vi "Aquire HackRF.vi"() -> ()   [LabVIEW 2020]
uses:
  <vilib>/sound2/lvsound2.llb/Sampling Mode.ctl
  <vilib>/sound2/lvsound2.llb/Sound Data Format.ctl
  <vilib>/Analysis/2dsp.llb/Decimate (single shot, DBL).vi
  <vilib>/addons/Adaptive Filters/Create/AFT Create FIR LMS (Real).vi
  <vilib>/addons/Digital Filter Design/Design.llb/DFD IIR Notch Peak Design by Q.vi
  <vilib>/sound2/lvsound2.llb/Sound Output Write (DBL Single).vi
  <vilib>/Analysis/3filter.llb/Butterworth Filter (CDB).vi
  <vilib>/measure/maresamp.llb/Resample Waveform (single shot).vi
  <vilib>/measure/maspectr.llb/FFT Spectrum (Mag-Phase) for 1 Chan.vi
  <vilib>/Analysis/3filter.llb/Butterworth Filter (DBL).vi
  <vilib>/Analysis/3filter.llb/IIR Filter (DBL).vi
  <vilib>/addons/Adaptive Filters/Processing/AFT Filter Signal and Update Coefficients (Real, Array).vi
  HRF_Device/HRF_Device.lvclass
  <vilib>/measure/NI_MAPro.lvlib
  <vilib>/Analysis/NI_AALBase.lvlib
  <vilib>/measure/NI_MABase.lvlib
  <vilib>/Analysis/NI_AALPro.lvlib
  <vilib>/addons/Adaptive Filters/NI_AdaptiveFilter.lvlib
  <vilib>/addons/Digital Filter Design/NI_DigFilterLicensed.lvlib
panel:
  in  "averaging parameters":T1={"averaging mode"=enum."Peak hold", "weighting mode"=enum."Linear", "number of averages"=10} {"number of averages" min=1}
  in  "view":T2={"dB On (F)"=TRUE, "unwrap phase (F)"=FALSE, "convert to degree (F)"=FALSE}
  in  "Enum 2":T3(ring)
  in  "sample rate (S/s)":enum16{"11025", "22050", "44100", "8000"}(ring)=enum."44100"
  in  "bits per sample":enum16{"8 bit", "16 bit"}(ring)=enum."16 bit"
  in  "channel":enum16{"mono", "stereo"}(ring)=enum."stereo"
  in  "scale":dbl=2.5 format="%#_13g"
  in  "cutoff freq":dbl=50000.0
  in  "order":i32=5
  in  "Enum":T3(ring)
  in  "Sample rate":dbl=44100.0
  in  "Interpolation mode":T4(ring)=enum."FIR filter"
  in  "Interpolation mode":T4(ring)=enum."FIR filter"
  in  "FIR filter specifications":T5={"alias rejection"=80.0, "norm bandwdt"=0.45}
  in  "FIR filter specifications":T5={"alias rejection"=40.0, "norm bandwdt"=0.45}
  in  "Resample":bool
  in  "Volume":dbl(knob)=0.76 step=0.01 scale=0.0..2.0
  in  "Order":i32=5
  in  "high cutoff freq: fh 2":dbl=100000.0 format="%0.2f"
  in  "filter input":bool=TRUE
  in  "averaging":bool=TRUE
  out "decimating factor":i32=5
  in  "Cutoff freq":dbl=50000.0 format="%#_13g"
  in  "Samples":dbl=200000.0 format="%#_13g"
  in  "frequency":dbl=10.0 format="%0.2p"
  in  "Q factor":dbl=20.0 format="%.2f"
  in  "f0 [Hz]":dbl=0.1 format="%.2f"
  in  "Scaling":dbl=0.008 format="%#_13g"
  in  "Boolean":bool
  in  "step size":dbl=0.01
  in  "shape":enum16{"rectangular", "triangular"}(ring)=enum."triangular"
  in  "type":enum16{"moving average", "exponential"}(ring)
  in  "half-width":i32=3
  out "df":dbl=inf
  in  "update":bool
  in  "shift":bool
  out "Backlog":u8(slide) scale=0.0..100.0
  in  "Resampling type":bool
  in  "averaging 2":bool=TRUE
  in  "decimating factor 2":i32=6
  out "spectral plot":cluster{"t":dbl, "t":dbl, "magnitude":dbl[]}(graph)={"t"=0.0, "t"=inf, "magnitude"=[]}
  out "Incoming":cluster{"t":dbl, "t":dbl, "magnitude":dbl[]}(graph)={"t"=0.0, "t"=1000000.0, "magnitude"=[-inf]}
  in  "Center freq":dbl=50000.0
  in  "LNA Gain dB":dbl(knob)=50.0 scale=0.0..50.0
  out "Resample Rate (dt)":dbl=2.2675736961451248e-05
  out "x-y 2":u32=328
  out "x-y":u32=525
  out "S/s":dbl(knob)=1000000.0 scale=0.0..5.0
  out "error out":errorcluster
  in  "Buffer size":i32=1000000
  in  "stop":bool
  in  "Filter Bandwidth":dbl(knob)=2.0 scale=0.0..1.0
  in  "TVA Gain dB":dbl(knob)=22.0 scale=0.0..50.0
  in  "Sample frequency":dbl(knob)=1.0 scale=0.0..5.0
  in  "Carrier frequency":dbl(knob)=101.1 step=0.01 scale=0.0..1000.0
  # "MS/sec"
  # "INPUT"
  # "FILTER"
  # "OUTPUT"
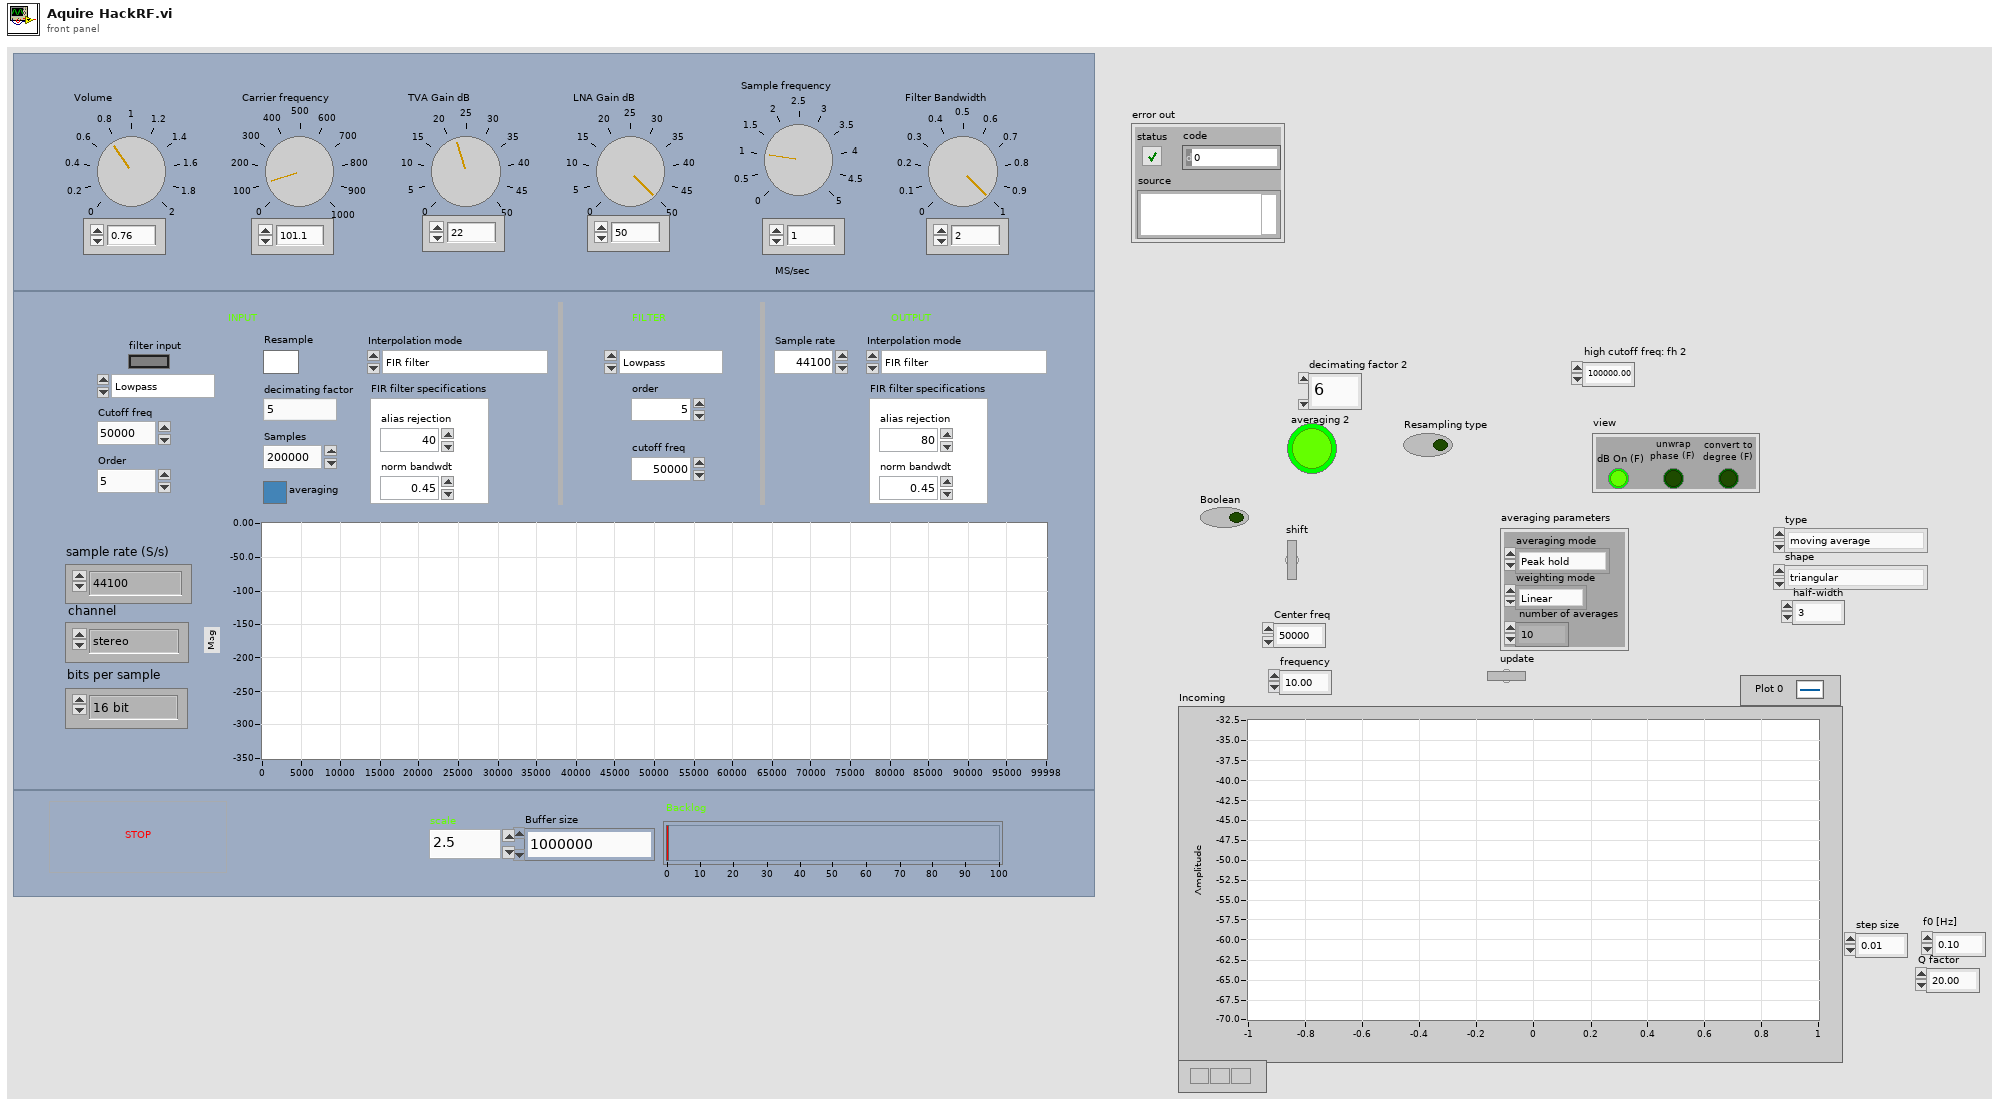
[diagram p1: front panel]
types:
  T1 = cluster{"averaging mode":enum16{"No averaging", "Vector averaging", "RMS averaging", "Peak hold"}, "weighting mode":enum16{"Linear", "Exponential"}, "number of averages":u32}
  T2 = cluster{"dB On (F)":bool, "unwrap phase (F)":bool, "convert to degree (F)":bool}
  T3 = enum16{"Lowpass", "Highpass", "Bandpass", "Bandstop"}
  T4 = enum16{"Coerce", "Linear", "Spline", "FIR filter"}
  T5 = cluster{"alias rejection":dbl, "norm bandwdt":dbl}
  T6 = cluster{"channel":enum16{"mono", "stereo"}, "sample rate (S/s)":enum16{"11025", "22050", "44100", "8000"}, "bits per sample":enum16{"8 bit", "16 bit"}}
  T7 = typedef "Sound Data Format.ctl" = cluster{"sample rate (S/s)":dbl, "number of channels":i32, "bits per sample":i32}
  T8 = typedef "Sampling Mode.ctl" = i32
  T9 = typedef "Sound Output Task ID.ctl" = u32
  T10 = enum16{"Sine Wave", "Triangle Wave", "Square Wave", "Sawtooth Wave"}
  T11 = typedef "NI_DigFilterLicensed.lvlib/DFD Filter Obj.ctl" = cluster{"mSRate_Fs":dbl, "mSRate_Version":string, "mSRate_Comments":string, "mSRate_OrgCoef":T12, "mSRate_CurCoef":T12, "mSRate_Quantized?":bool, "mSRate_QCoef":T12, "mSRate_QSettings":T14[], "mSRate_Order":i32, "mSRate_Scaling":cluster{"mSRate_ScaleByPowerOf2?":bool, "mSRate_ScaleType":T16}}
  T12 = typedef "NI_DigFilterLicensed.lvlib/DFD Filter Coef.ctl" = cluster{"type":T13, "gain":dbl, "coef a (k)":dbl[], "coef b (v)":dbl[]}
  T13 = typedef "NI_DigFilterLicensed.lvlib/DFD Filter Structure Type Selector.ctl" = enum16{"Undefined", "FIR Direct Form", "FIR Direct Form Transposed", "FIR Symmetric", "FIR Antisymmetric", "IIR Direct Form I", "IIR Direct Form I Transposed", "IIR Direct Form II", "IIR Direct Form II Transposed", "IIR Cascaded Second Order Sections Form I", "IIR Cascaded Second Order Sections Form I Transposed", "IIR Cascaded Second Order Sections Form II", "IIR Cascaded Second Order Sections Form II Transposed", "Lattice Allpass (basic sections)", "Lattice Allpass (one multiplier sections)", "Lattice Allpass (normalized sections)", "Lattice AR (basic sections)", "Lattice AR (one multiplier sections)", "Lattice AR (normalized sections)", "Lattice MA (minimum phase)", "Lattice MA (maximum phase)", "Lattice ARMA (basic sections)", "Lattice ARMA (one multiplier sections)", "Lattice ARMA (normalized sections)"}
  T14 = typedef "NI_DigFilterLicensed.lvlib/dfd_Internal Quantization Settings.ctl" = cluster{"source":T15, "wl":i16, "iwl":i16, "overflow mode":enum16{"Saturation", "Wrap"}, "rounding mode":enum16{"Nearest", "Truncation"}, "signed?":bool}
  T15 = typedef "NI_DigFilterLicensed.lvlib/dfd_Internal Quantization Srcs.ctl" = u16
  T16 = typedef "NI_DigFilterLicensed.lvlib/DFD Coef Norm Type.ctl" = enum16{"No Norm", "Time Domain 1-Norm", "Time Domain 2-Norm", "Time Domain Inf-Norm"}
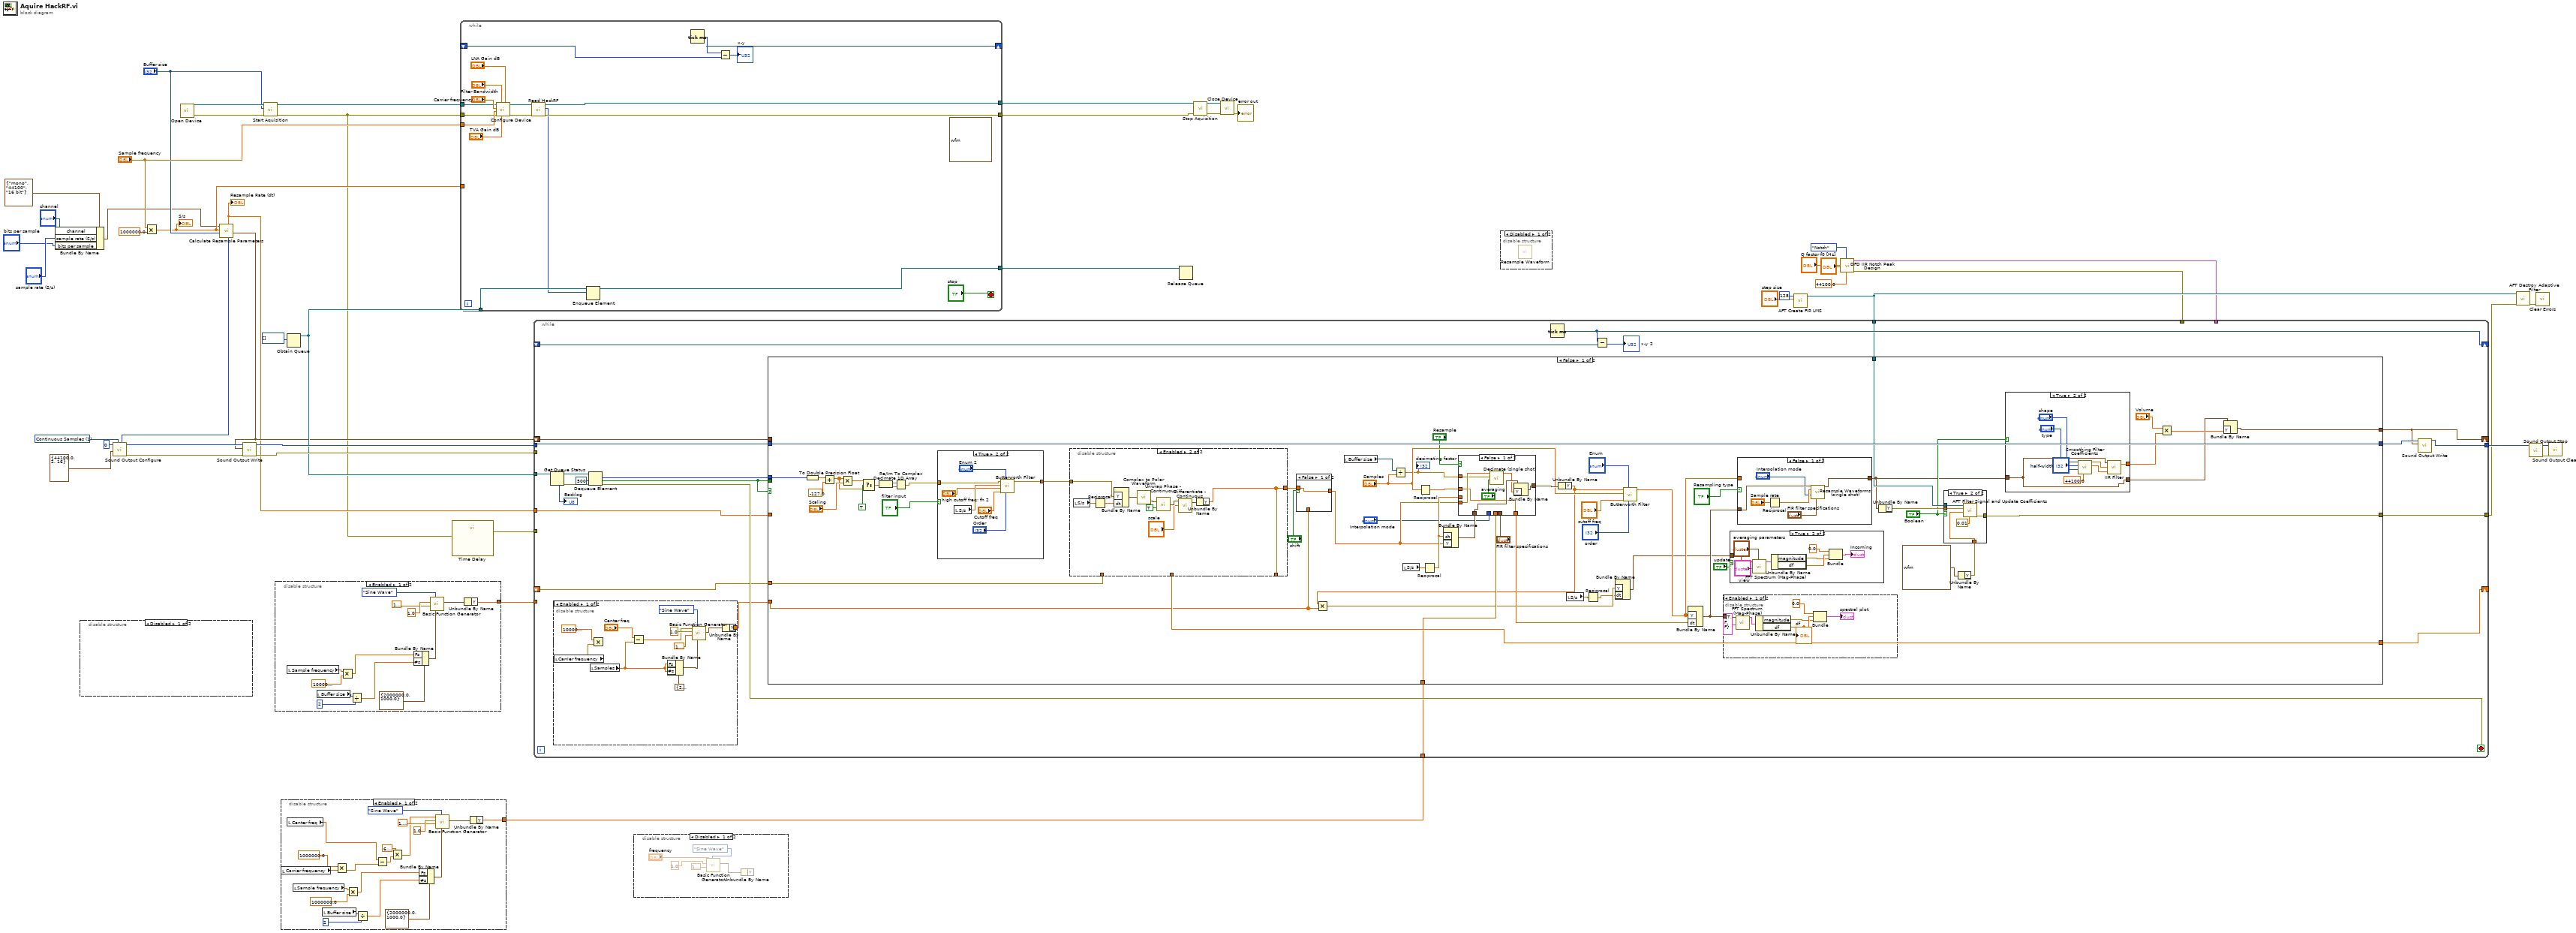
[diagram p0: block diagram]
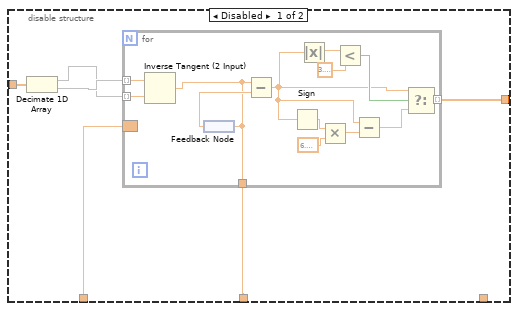
[diagram p8: hidden frame]
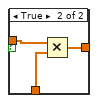
[diagram p9: hidden frame]
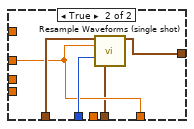
[diagram p10: hidden frame]
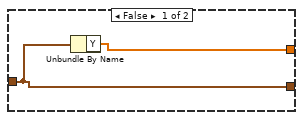
[diagram p12: hidden frame]
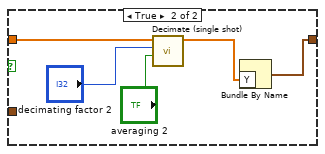
[diagram p15: hidden frame]
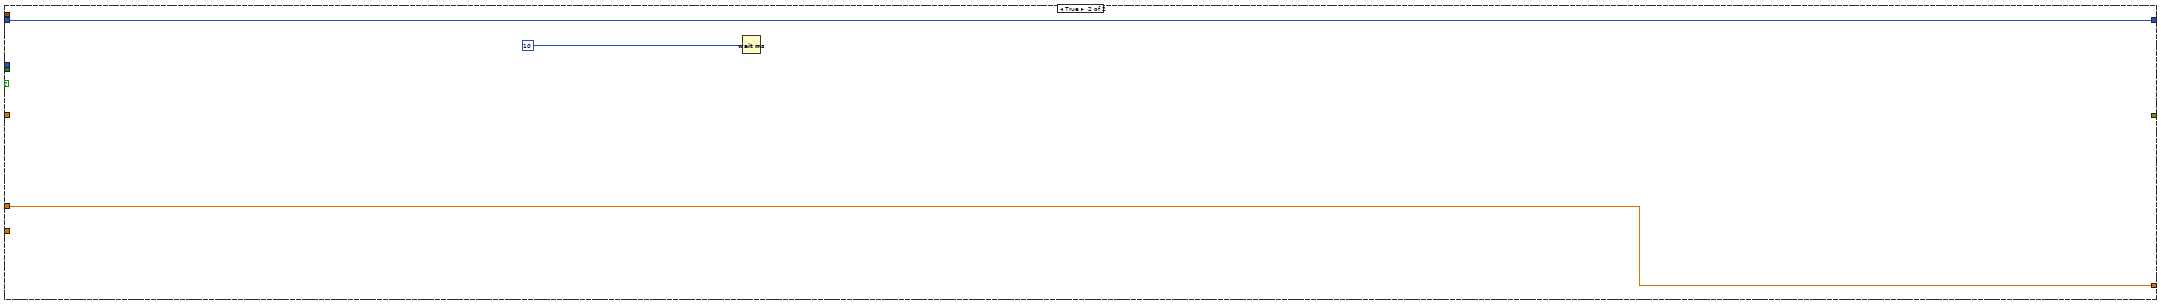
[diagram p17: hidden frame]
diagram:
  w41 = T8 1 items=["Finite Samples", "Continuous Samples"] ("sample mode")
  n1 = Bundle By Name(cluster=T6 {"channel"=enum."mono", "sample rate (S/s)"=enum."44100", "bits per sample"=enum."16 bit"} ("Sound Format"), "channel"="channel", "sample rate (S/s)"="sample rate (S/s)", "bits per sample"="bits per sample") -> (w1:T6)
  n2 = disable-structure shown="Disabled" {
    frame Disabled {
    }
    frame Enabled {
    }
  }
  n3 = Multiply(x="Sample frequency", y=1000000.0) -> (x*y=w27:dbl)
  "S/s" <- w27
  n4 = call "Open Device.vi"() -> ("error out"=w29:errorcluster, "HRF_Device out"=w30:refnum<class "HRF_Device.lvclass">)  [unwired: 10 in]
  n5 = call "Calculate Resample Parameters.vi"("Original Frame Size (Samples)"="Buffer size", "Original Sample Rate (S/s)"=w27, "Sound Format"=w1) -> ("Audio Waveform Init"=w22:waveform(dbl), "Resample Buffer Size (Samp)"=w23:i32, "Resample Rate (dt)"=w21:dbl)  [unwired: 5 in, 1 out]
  "Resample Rate (dt)" <- w21
  n6 = call <vilib>:"Sound Output Configure.vi"("number of samples/ch"=w23, "sample mode"=w41, "sound format"=T7 {"sample rate (S/s)"=44100.0, "number of channels"=2, "bits per sample"=16} ("Sound Format"), "device ID"=u32 0) -> ("error out"=w39:errorcluster, "task ID"=w40:T9)  [unwired: 6 in]
  n7 = call-poly <vilib>:"Sound Output Write.vi"("error in (no error)"=w39, "data"=w22, "task ID"=w40) -> ("error out"=w32:errorcluster, "task ID out"=w34:T9)  [unwired: 7 in]
  n8 = call "Start Aquisition.vi"("error in (no error)"=w29, "Buffer size"="Buffer size", "HRF_Device"=w30) -> ("error out"=w19:errorcluster, "HRF_Device"=w48:refnum<class "HRF_Device.lvclass">)  [unwired: 7 in]
  n9 = disable-structure shown="Enabled" {
    disable-tunnel: [w52 _] -> w18
    frame Enabled {
      n10 = local read "Sample frequency"() -> (w55:dbl)
      n11 = local read "Buffer size"() -> (w51:i32)
      n12 = Multiply(x=w55, y=1000000.0 ("x")) -> (x*y=w53:dbl)
      n13 = Divide(x=w51, y=2) -> (x/y=w50:dbl)
      n14 = Bundle By Name(cluster=cluster{"Fs":dbl, "#s":dbl} {"Fs"=2000000.0, "#s"=1000.0} ("sampling info"), "Fs"=w53, "#s"=w50) -> (w58:cluster{"Fs":dbl, "#s":dbl})
      n15 = call <vilib>:"Basic Function Generator.vi"("sampling info"=w58, "signal type"=T10."Sine Wave", "phase"=1.5707963267948966, "amplitude"=1.0) -> ("signal out"=w56:waveform(dbl))  [unwired: 5 in, 2 out]
      n16 = Unbundle By Name(w56) -> ("Y"=w52:dbl[])
    }
    frame Disabled {
    }
  }
  n17 = disable-structure shown="Enabled" {
    disable-tunnel: [w69 _] -> w17
    frame Enabled {
      n18 = local read "Carrier frequency"() -> (w77:dbl)
      n19 = local read "Center freq"() -> (w65:dbl)
      n20 = local read "Sample frequency"() -> (w72:dbl)
      n21 = local read "Buffer size"() -> (w68:i32)
      n22 = Multiply(x=1000000.0, y=w77) -> (x*y=w74:dbl)
      n23 = Multiply(x=w72, y=1000000.0 ("x")) -> (x*y=w70:dbl)
      n24 = Divide(x=w68, y=2) -> (x/y=w67:dbl)
      n25 = Subtract(x=w65, y=w74) -> (x-y=w64:dbl)
      n26 = Multiply(x=6.283185307179586, y=w64) -> (x*y=w62:dbl)
      n27 = Bundle By Name(cluster=cluster{"Fs":dbl, "#s":dbl} {"Fs"=2000000.0, "#s"=1000.0} ("sampling info"), "Fs"=w70, "#s"=w67) -> (w78:cluster{"Fs":dbl, "#s":dbl})
      n28 = call <vilib>:"Basic Function Generator.vi"("sampling info"=w78, "signal type"=T10."Sine Wave", "phase"=1.5707963267948966, "amplitude"=1.0, "frequency"=w62) -> ("signal out"=w75:waveform(dbl))  [unwired: 4 in, 2 out]
      n29 = Unbundle By Name(w75) -> ("Y"=w69:dbl[])
    }
    frame Disabled {
    }
  }
  n30 = Obtain Queue(element data type=u8[] []) -> (queue out=w24:refnum<queue>)  [unwired: 4 in, 2 out]
  n31 = call "Time Delay"("error in (no error)"=w19) -> ("error out"=w20:errorcluster)  [unwired: 10 in]
  n32 = while {
    tunnel: w19 -> [w92]
    tunnel: w48 -> [w91]
    tunnel: [w98] -> w47
    tunnel: [w97] -> w46
    tunnel: w27 -> [_]
    tunnel: "Sample frequency" -> [w93]
    shift-right: [w88] -> _
    shift-left: _ -> [w87]
    tunnel: w24 -> [w85]
    tunnel: [w83] -> w25
    stop <- "stop" stop-if-true
    (unwired) waveform(cdb) {"t0"=timestamp(0 s since 1904-01-01), "dt"=1.0, "Y"=[]} ("IQ Waveform Init")
    n33 = call "Configure Device.vi"("LNA Gain dB"="LNA Gain dB", "TVA Gain dB"="TVA Gain dB", "Filter Bandwidth"="Filter Bandwidth", "error in (no error)"=w92, "Sample frequency"=w93, "Carrier frequency"="Carrier frequency", "HRF_Device"=w91) -> ("error out"=w89:errorcluster, "HRF_Device"=w90:refnum<class "HRF_Device.lvclass">)  [unwired: 3 in]
    n34 = call "Read HackRF.vi"("error in (no error)"=w89, "HRF_Device"=w90) -> ("error out"=w98:errorcluster, "Array"=w84:u8[], "HRF_Device out"=w97:refnum<class "HRF_Device.lvclass">)  [unwired: 7 in]
    n35 = Enqueue Element(queue=w85, element=w84) -> (queue out=w83:refnum<queue>)  [unwired: 2 in, 2 out]
    n36 = Tick Count (ms)() -> (millisecond timer value=w88:u32)
    n37 = Subtract(x=w88, y=w87) -> (x-y=→"x-y":u32)
  }
  n38 = disable-structure shown="Disabled" {
    frame Disabled {
      n39 = call <vilib>:"Basic Function Generator.vi"("signal type"=T10."Sine Wave", "phase"=1.5707963267948966, "amplitude"=1.0, "frequency"="frequency") -> ("signal out"=w104:waveform(dbl))  [unwired: 5 in, 2 out]
      n40 = Unbundle By Name(w104) -> ()  [unwired: 1 out]
    }
    frame Enabled {
    }
  }
  n41 = Release Queue(queue=w25) -> ()  [unwired: 2 in, 3 out]
  n42 = call "Stop Aquisition.vi"("error in (no error)"=w47, "HRF_Device"=w46) -> ("error out"=w45:errorcluster, "HRF_Device"=w44:refnum<class "HRF_Device.lvclass">)  [unwired: 8 in]
  n43 = call "Close Device.vi"("error in (no error)"=w45, "HRF_Device"=w44) -> ("error out"=→"error out":errorcluster)  [unwired: 9 in]
  n44 = disable-structure shown="Disabled" {
    frame Disabled {
      n45 = call "Resample Waveform.vi"() -> ()  [unwired: 12 in, 4 out]
    }
    frame Enabled {
    }
  }
  n46 = call-poly <vilib>:"AFT Create FIR LMS.vi"("step size"="step size", "filter length"=128) -> ("adaptive filter out"=w14:refnum<k20>)  [unwired: 2 in, 7 out]
  n47 = call-poly <vilib>:"DFD IIR Notch Peak Design.vi"("fs [Hz]"=44100.0 ("fs"), "filter type"=enum16{"Notch", "Peak"}."Notch", "Q factor"="Q factor", "f0 [Hz]"="f0 [Hz]") -> ("error out"=w6:errorcluster, "filter out"=w7:T11)  [unwired: 6 in]
  n48 = while {
    tunnel: w34 -> [w122]
    tunnel: [w112] -> w33
    tunnel: w32 -> [_]
    shift-right: [w127] -> _
    shift-left: _ -> [w126]
    tunnel: w24 -> [w124]
    tunnel: w21 -> [w119]
    shift-right: [w113] -> _
    shift-left: w22 -> [w120]
    shift-right: [w117] -> _
    shift-left: _ -> [w116]
    tunnel: w20 -> [_]
    tunnel: w18 -> [_]
    tunnel: w17 -> [w108]
    tunnel: w14 -> [w107]
    tunnel: [w106] -> w13
    tunnel: w7 -> [_]
    tunnel: w6 -> [_]
    stop <- w123 stop-if-true
    n49 = Get Queue Status(queue=w124) -> (queue out=w111:refnum<queue>, error out=w109:errorcluster, # elements in queue=→"Backlog":i32)  [unwired: 2 in, 5 out]
    n50 = disable-structure shown="Enabled" {
      disable-tunnel: [w132 _] -> w105
      frame Enabled {
        n51 = local read "Carrier frequency"() -> (w136:dbl)
        n52 = local read "Samples"() -> (w128:dbl)
        n53 = Multiply(x=1000000.0, y=w136) -> ()  [unwired: 1 out]
        n54 = Subtract(x="Center freq", y=w128) -> (x-y=w129:dbl)
        n55 = Bundle By Name(cluster=cluster{"Fs":dbl, "#s":dbl} {"Fs"=2000000.0, "#s"=1000.0} ("sampling info"), "Fs"=w128, "#s"=w128) -> (w130:cluster{"Fs":dbl, "#s":dbl})
        n56 = call <vilib>:"Basic Function Generator.vi"("sampling info"=w130, "signal type"=T10."Sine Wave", "phase"=1.5707963267948966, "amplitude"=1.0, "frequency"=w129) -> ("signal out"=w133:waveform(dbl))  [unwired: 4 in, 2 out]
        n57 = Unbundle By Name(w133) -> ("Y"=w132:dbl[])
      }
      frame Disabled {
      }
    }
    n58 = Dequeue Element(queue=w111, timeout in ms (-1)=500, error in (no error)=w109) -> (element=w121:u8[], timed out?=w115:bool, error out=w123:errorcluster)  [unwired: 1 out]
    n59 = case shown="False" w115 {
      tunnel: [w195 w291] -> w114
      tunnel: [w196 _] -> w113
      tunnel: w122 -> [w195 w291]
      tunnel: w121 -> [w194 _]
      tunnel: w120 -> [_ _]
      tunnel: w115 -> [_ _]
      tunnel: w119 -> [_ _]
      tunnel: [w193 w293] -> w117
      tunnel: w116 -> [w192 w293]
      tunnel: w105 -> [w145 _]
      tunnel: w108 -> [w191 _]
      tunnel: w107 -> [w190 _]
      tunnel: [w189 _] -> w106
      frame False {
        n60 = To Double Precision Float(number=w194) -> (double precision float=w188:dbl[])
        n61 = Add(x=w188, y=-127.0 ("Numeric")) -> (x+y=w179:dbl[])
        n62 = Multiply(x=w179, y="Scaling") -> (x*y=w180:dbl[])
        n63 = Select(t=w180, s=TRUE ("scale"), f=w179) -> (s? t:f=w149:dbl[])
        n64 = Decimate 1D Array(w149) -> (w148:dbl[], w147:dbl[])
        n65 = Re/Im To Complex(1:w147, 2:w148) -> (0:w146:cdb[])
        n66 = case shown="True" "filter input" {
          tunnel: w146 -> [w242 w245]
          tunnel: [w242 w244] -> w168
          frame False {
          }
          frame True {
            n67 = local read "S/s"() -> (w248:dbl)
            n68 = call-poly <vilib>:"Butterworth Filter.vi"("order"="Order", "filter type"="Enum 2", "low cutoff freq: fl"="Cutoff freq", "high cutoff freq: fh"="high cutoff freq: fh 2", "sampling freq: fs"=w248, "X"=w245) -> ("Filtered X"=w244:cdb[])  [unwired: 2 in, 1 out]
          }
        }
        n69 = disable-structure shown="Enabled" {
          disable-tunnel: [w202 _] -> w193
          disable-tunnel: w192 -> [w201 _]
          disable-tunnel: w168 -> [w200 w217]
          disable-tunnel: [w197 w216] -> w158
          disable-tunnel: [_ w216] -> _
          frame Disabled {
            n70 = Decimate 1D Array(w200) -> (w198:cdb[], w199:cdb[])
            n71 = for {
              tunnel: [w208] -> w197 mode=indexing
              tunnel: w199 -> [w207] mode=indexing
              tunnel: w198 -> [w206] mode=indexing
              border: w201 -> [_]
              tunnel: [w204] -> w202
              n72 = Inverse Tangent (2 Input)(1:w206, 2:w207) -> (0:w204:cdb)
              n73 = feedback #1() -> (w205:cdb)
              n74 = feedback-in #1(w204) -> ()
              n75 = Subtract(x=w204, y=w205) -> (x-y=w203:cdb)
              n76 = Sign(1:w203) -> (0:w215:cdb)
              n77 = Absolute Value(x=w203) -> (abs(x)=w211:dbl)
              n78 = Multiply(x=w215, y=6.283185307179586) -> (x*y=w213:cdb)
              n79 = Less?(x=w211, y=3.141592653589793) -> (x < y?=w209:bool)
              n80 = Subtract(x=w203, y=w213) -> (x-y=w212:cdb)
              n81 = Select(t=w203, s=w209, f=w212) -> (s? t:f=w208:cdb)
            }
          }
          frame Enabled {
            n82 = local read "S/s"() -> (w225:dbl)
            n83 = Reciprocal(x=w225) -> (1/x=w224:dbl)
            n84 = Bundle By Name("Y"=w217, "dt"=w224) -> (w223:waveform(cdb))  [unwired: 1 in]
            n85 = call "Complex to Polar Waveform.vi"("Input Signal"=w223) -> ("Angle"=w222:waveform(dbl))  [unwired: 1 out]
            n86 = call "Unwrap Phase - Continuous.vi"("Reset"=TRUE, "Input Signal"=w222) -> ("Phase Unwrapped"=w221:waveform(dbl))
            n87 = call "Differentiate - Continuous.vi"("dx/dt 2"="scale", "Input Signal"=w221) -> ("dx/dt"=w220:waveform(dbl))  [unwired: 2 in]
            n88 = Unbundle By Name(w220) -> ("Y"=w216:dbl[])
          }
        }
        n89 = case shown="False" "shift" {
          tunnel: [w226 w229] -> w154
          tunnel: w158 -> [w226 w228]
          tunnel: w145 -> [_ w227]
          frame False {
          }
          frame True {
            n90 = Multiply(x=w228, y=w227) -> (x*y=w229:dbl[])
          }
        }
        n91 = local read "Buffer size"() -> (w151:i32)
        n92 = Divide(x=w151, y="Samples") -> (x/y=w150:dbl)
        "decimating factor" <- w150
        n93 = local read "S/s"() -> (w159:dbl)
        n94 = Reciprocal(x="Samples") -> (1/x=w155:dbl)
        n95 = Reciprocal(x=w159) -> (1/x=w156:dbl)
        n96 = Bundle By Name("dt"=w156, "Y"=w154) -> (w183:waveform(dbl))  [unwired: 1 in]
        n97 = case shown="False" "Resample" {
          tunnel: w183 -> [w235 w240]
          tunnel: [w233 w241] -> w173
          tunnel: w155 -> [w231 w238]
          tunnel: "Interpolation mode" -> [_ w239]
          tunnel: [w231 w238] -> w174
          tunnel: w191 -> [_ _]
          tunnel: w156 -> [_ _]
          tunnel: w154 -> [w236 _]
          tunnel: "FIR filter specifications" -> [_ w237]
          tunnel: w150 -> [w230 _]
          frame False {
            n98 = call-poly <vilib>:"Decimate (single shot).vi"("averaging"="averaging", "decimating factor"=w230, "X"=w236) -> ("Decimated Array"=w234:dbl[])  [unwired: 7 in, 1 out]
            n99 = Bundle By Name(cluster=w235, "Y"=w234) -> (w233:waveform(dbl))
          }
          frame True {
            n100 = call-poly <vilib>:"Resample Waveforms (single shot).vi"("waveform in"=w240, "dt"=w238, "interpolation mode"=w239, "FIR filter specifications"=w237) -> ("resampled waveform out"=w241:waveform(dbl))  [unwired: 8 in, 3 out]
          }
        }
        n101 = Unbundle By Name(w173) -> ("Y"=w140:dbl[])
        n102 = Multiply(x=w140, y=w145) -> (x*y=w144:dbl[])
        n103 = local read "S/s"() -> (w143:dbl)
        n104 = Reciprocal(x=w143) -> (1/x=w142:dbl)
        n105 = Bundle By Name("Y"=w144, "dt"=w142) -> (w141:waveform(dbl))  [unwired: 1 in]
        n106 = call-poly <vilib>:"Butterworth Filter.vi"("order"="order", "filter type"="Enum", "low cutoff freq: fl"="cutoff freq", "sampling freq: fs"="Samples", "X"=w140) -> ("Filtered X"=w169:dbl[])  [unwired: 3 in, 1 out]
        n107 = Bundle By Name("Y"=w169, "dt"=w174) -> (w171:waveform(dbl))  [unwired: 1 in]
        n108 = disable-structure shown="Enabled" {
          disable-tunnel: w171 -> [w285 _]
          frame Enabled {
            n109 = call-poly <vilib>:"FFT Spectrum (Mag-Phase).vi"("view"=T2 {"dB On (F)"=TRUE, "unwrap phase (F)"=FALSE, "convert to degree (F)"=FALSE}, "time signal"=w285) -> ("magnitude"=w290:cluster{"f0":dbl, "df":dbl, "magnitude":dbl[]})  [unwired: 5 in, 4 out]
            n110 = Unbundle By Name(w290) -> ("magnitude"=w286:dbl[], "df"=w287:dbl)
            "df" <- w287
            n111 = Bundle(0.0, "df"=w287, "magnitude"=w286) -> (→"spectral plot":cluster{dbl, "df":dbl, "magnitude":dbl[]})  [unwired: 1 in]
          }
          frame Disabled {
          }
        }
        n112 = case shown="True" "update" {
          tunnel: w141 -> [_ w267]
          frame False {
          }
          frame True {
            n113 = call-poly <vilib>:"FFT Spectrum (Mag-Phase).vi"("averaging parameters"="averaging parameters", "view"="view", "time signal"=w267) -> ("magnitude"=w272:cluster{"f0":dbl, "df":dbl, "magnitude":dbl[]})  [unwired: 4 in, 4 out]
            n114 = Unbundle By Name(w272) -> ("magnitude"=w269:dbl[], "df"=w270:dbl)
            n115 = Bundle(0.0, "df"=w270, "magnitude"=w269) -> (→"Incoming":cluster{dbl, "df":dbl, "magnitude":dbl[]})  [unwired: 1 in]
          }
        }
        n116 = case shown="False" "Resampling type" {
          tunnel: [w276 w280] -> w172
          tunnel: w169 -> [_ w281]
          tunnel: w171 -> [w277 _]
          frame False {
            n117 = Reciprocal(x="Sample rate") -> (1/x=w278:dbl)
            n118 = call-poly <vilib>:"Resample Waveforms (single shot).vi"("waveform in"=w277, "dt"=w278, "interpolation mode"="Interpolation mode", "FIR filter specifications"="FIR filter specifications") -> ("resampled waveform out"=w276:waveform(dbl))  [unwired: 8 in, 3 out]
          }
          frame True {
            n119 = call-poly <vilib>:"Decimate (single shot).vi"("averaging"="averaging 2", "decimating factor"="decimating factor 2", "X"=w281) -> ("Decimated Array"=w279:dbl[])  [unwired: 7 in, 1 out]
            n120 = Bundle By Name("Y"=w279) -> (w280:waveform(dbl))  [unwired: 1 in]
          }
        }
        n121 = Unbundle By Name(w172) -> ("Y"=w182:dbl[])
        n122 = Unbundle By Name(waveform(dbl) {"t0"=timestamp(0 s since 1904-01-01), "dt"=2.2675736961451248e-05, "Y"=array[22050 elements]} ("resampled waveform out")) -> ("Y"=w177:dbl[])
        n123 = case shown="True" "Boolean" {
          tunnel: w190 -> [_ w264]
          tunnel: w182 -> [_ w263]
          tunnel: [_ w262] -> w189
          tunnel: w177 -> [_ w260]
          frame False {
          }
          frame True {
            n124 = call-poly <vilib>:"AFT Filter Signal and Update Coefficients.vi"("step size"=0.01, "d(n)"=w260, "x(n)"=w263, "adaptive filter in"=w264) -> ("error out"=w262:errorcluster)  [unwired: 2 in, 5 out]
          }
        }
        n125 = case shown="True" "Boolean" {
          tunnel: w172 -> [w250 w252]
          tunnel: [w251 w259] -> w176
          tunnel: [w250 w252] -> w165
          frame False {
            n126 = Unbundle By Name(w250) -> ("Y"=w251:dbl[])
          }
          frame True {
            n127 = call <vilib>:"Smoothing Filter Coefficients.vi"("fs"=44100.0, "shape"="shape", "half-width"="half-width", "type"="type") -> ("forward coefficients"=w257:dbl[], "reverse coefficients"=w258:dbl[])  [unwired: 5 in, 1 out]
            n128 = call-poly <vilib>:"IIR Filter.vi"("Forward Coefficients"=w257, "Reverse Coefficients"=w258, "X"=w252) -> ("Filtered X"=w259:dbl[])  [unwired: 1 in, 1 out]
          }
        }
        n129 = Multiply(x="Volume", y=w176) -> (x*y=w166:dbl[])
        n130 = Bundle By Name(cluster=w165, "Y"=w166) -> (w196:waveform(dbl))
      }
      frame True {
        n131 = Wait (ms)(milliseconds to wait=u32 10) -> ()  [unwired: 1 out]
      }
    }
    n132 = Tick Count (ms)() -> (millisecond timer value=w127:u32)
    n133 = Subtract(x=w127, y=w126) -> (x-y=→"x-y 2":u32)
    n134 = call-poly <vilib>:"Sound Output Write.vi"("data"=w113, "task ID"=w114) -> ("task ID out"=w112:T9)  [unwired: 8 in, 1 out]
  }
  n135 = call <vilib>:"AFT Destroy Adaptive Filter.vi"("error in (no error)"=w13, "adaptive filter in"=w14) -> ("error out"=w12:errorcluster)  [unwired: 9 out]
  n136 = call <vilib>:"Sound Output Stop.vi"("task ID"=w33) -> ("error out"=w38:errorcluster, "task ID out"=w37:T9)  [unwired: 9 in]
  n137 = call <vilib>:"Clear Errors.vi"("error in (no error)"=w12) -> ()  [unwired: 5 in, 2 out]
  n138 = call <vilib>:"Sound Output Clear.vi"("error in (no error)"=w38, "task ID"=w37) -> ()  [unwired: 9 in, 1 out]
